vi "clear_data_paths.vi"(8 "error in (no error)":errorcluster) -> (0 "error out":errorcluster)   [LabVIEW 2015, in "lv-bin.lvlib" / "v1.lvlib"]
uses:
  v1.lvlib
  private/_controls/fg_command.ctl
  lv-bin.lvlib
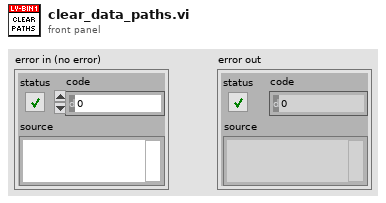
[diagram p1: front panel]
types:
  T1 = typedef "lv-bin.lvlib/fg_command.ctl" = enum16{"<fg_command>", "initialize", "read", "write", "shutdown", "<null>"}
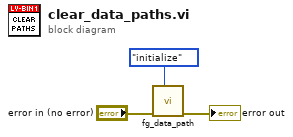
[diagram p0: block diagram]
diagram:
  n1 = call "fg_data_path.vi"("fg_command"=fg_command."initialize", "error in (no error)"="error in (no error)") -> ("error out"=→"error out":errorcluster)  [unwired: 8 in, 1 out]
